vi "KINECTcheckMusclesAngle.vi"(8 "Muscle Tolerance":dbl=0.25, 9 "Hand":cluster{"x":dbl, "y":dbl, "z":dbl}, 10 "Elbow":cluster{"x":dbl, "y":dbl, "z":dbl}, 11 "Shoulder":cluster{"x":dbl, "y":dbl, "z":dbl}) -> (3 "Go to Calibrate":bool)   [LabVIEW 2011]
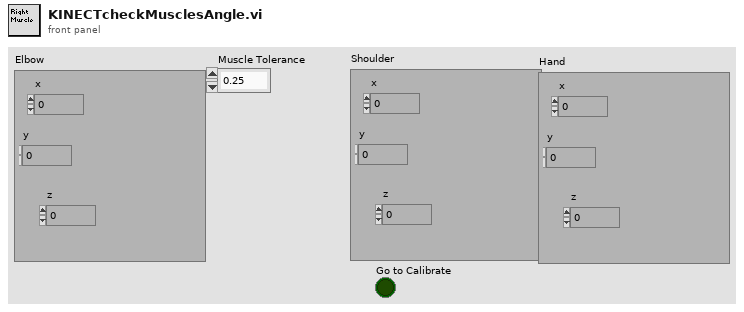
[diagram p1: front panel]
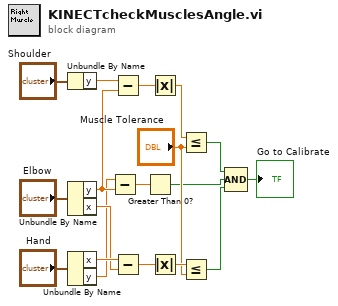
[diagram p0: block diagram]
diagram:
  n1 = Unbundle By Name("Shoulder") -> ("y"=w15:dbl)
  n2 = Unbundle By Name("Elbow") -> ("y"=w7:dbl, "x"=w13:dbl)
  n3 = Unbundle By Name("Hand") -> ("x"=w14:dbl, "y"=w6:dbl)
  n4 = Subtract(x=w6, y=w7) -> (x-y=w5:dbl)
  n5 = Subtract(x=w15, y=w7) -> (x-y=w10:dbl)
  n6 = Subtract(x=w14, y=w13) -> (x-y=w12:dbl)
  n7 = Greater Than 0?(x=w5) -> (x > 0?=w3:bool)
  n8 = Absolute Value(x=w10) -> (abs(x)=w9:dbl)
  n9 = Absolute Value(x=w12) -> (abs(x)=w11:dbl)
  n10 = Less Or Equal?(x=w9, y="Muscle Tolerance") -> (x <= y?=w4:bool)
  n11 = Less Or Equal?(x=w11, y="Muscle Tolerance") -> (x <= y?=w2:bool)
  n12 = Compound Arithmetic op=AND(w4, w3, w2) -> (→"Go to Calibrate":bool)
